vi "sameB.vi"(7 "B [T] new":dbl, 11 "B [T] old":dbl) -> (3 "Boolean":bool)   [LabVIEW 2013]
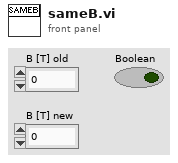
[diagram p1: front panel]
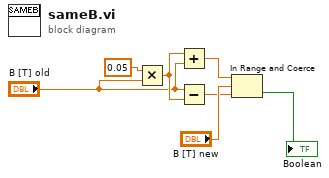
[diagram p0: block diagram]
diagram:
  n1 = Multiply(x=0.05, y="B [T] old") -> (x*y=w4:dbl)
  n2 = Add(x=w4, y="B [T] old") -> (x+y=w2:dbl)
  n3 = Subtract(x="B [T] old", y=w4) -> (x-y=w5:dbl)
  n4 = In Range and Coerce(upper limit=w2, x="B [T] new", lower limit=w5) -> (In Range?=→"Boolean":bool)  [unwired: 1 out]
